vi "Autonomous A2 left-deliverswitch-move out of way.vi"   [LabVIEW 2017]
uses:
  Framework/Robot Global Data.vi
types:
  T1 = typedef "Command Status Info.ctl" = cluster{"Name":string, "Status":T2, "notifier out":T3}
  T2 = typedef "Completion Status.ctl" = enum16{"Successful", "Aborted", "Incomplete"}
  T3 = typedef "Completion Notifier.ctl" = refnum<notifier>
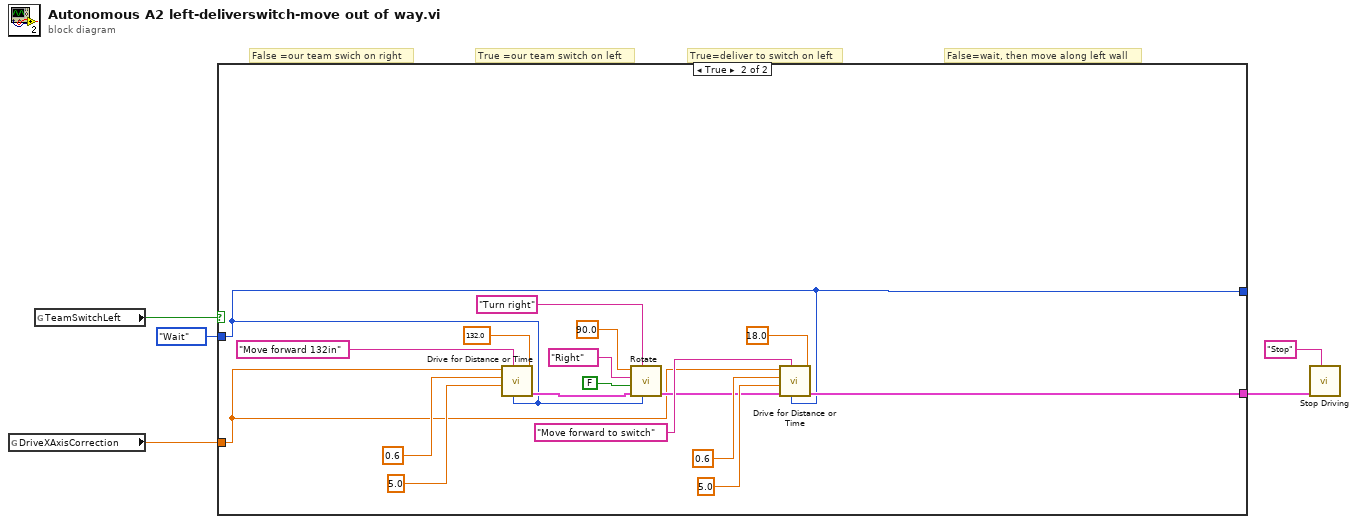
[diagram p0: block diagram]
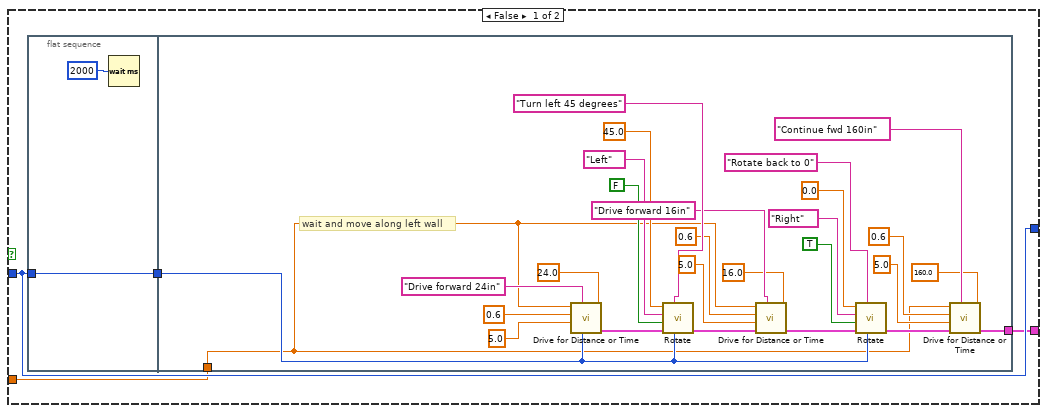
[diagram p2: hidden frame]
diagram:
  # "False=wait, then move along left wall"
  # "True=deliver to switch on left"
  # "False =our team swich on right"
  # "True =our team switch on left"
  n1 = global read "Robot Global Data.vi" "DriveXAxisCorrection"() -> (w1:dbl)
  n2 = global read "Robot Global Data.vi" "TeamSwitchLeft"() -> (w2:bool)
  n3 = case shown="True" w2 {
    tunnel: enum16{"Start", "Wait"}."Wait" ("Synchronication") -> [w9 w43]
    tunnel: [w7 w52] -> w3
    tunnel: [w9 w43] -> _
    tunnel: w1 -> [w6 w39]
    frame False {
      n4 = flat-sequence {
        tunnel: w9 -> [w11]
        tunnel: [w11] -> w8
        tunnel: w8 -> [w29]
        tunnel: [w15] -> w7
        tunnel: w6 -> [w12]
        frame #0 {
          n5 = Wait (ms)(milliseconds to wait=u32 2000) -> ()  [unwired: 1 out]
        }
        frame #1 {
          # "wait and move along left wall"
          n6 = call "Drive for Distance or Time.vi"("Distance (inches)"=24.0, "Synchronication"=w29, "Description"="Drive forward 24in", "Seconds"=5.0, "Y-axis"=0.6 ("Right Speed"), "X-axis"=w12) -> ("Command Info Out"=w35:T1)  [unwired: 5 in]
          n7 = call "Rotate.vi"("Synchronication"=w29, "Description"="Turn left 45 degrees", "Command Info In"=w35, "Force Degrees"=FALSE, "Turn Direction"="Left" ("Direction"), "Degrees"=45.0) -> ("Command Info Out"=w24:T1)  [unwired: 5 in]
          n8 = call "Drive for Distance or Time.vi"("Distance (inches)"=16.0, "Description"="Drive forward 16in", "Command Info In"=w24, "Seconds"=5.0, "Y-axis"=0.6 ("Right Speed"), "X-axis"=w12) -> ("Command Info Out"=w23:T1)  [unwired: 5 in]
          n9 = call "Rotate.vi"("Synchronication"=w29, "Description"="Rotate back to 0", "Command Info In"=w23, "Force Degrees"=TRUE, "Turn Direction"="Right" ("Direction"), "Degrees"=0.0 ("Seconds")) -> ("Command Info Out"=w22:T1)  [unwired: 5 in]
          n10 = call "Drive for Distance or Time.vi"("Distance (inches)"=160.0, "Description"="Continue fwd 160in", "Command Info In"=w22, "Seconds"=5.0, "Y-axis"=0.6, "X-axis"=w12) -> ("Command Info Out"=w15:T1)  [unwired: 5 in]
        }
      }
    }
    frame True {
      n11 = call "Drive for Distance or Time.vi"("Distance (inches)"=132.0, "Synchronication"=w43, "Description"="Move forward 132in", "Seconds"=5.0, "Y-axis"=0.6 ("Right Speed"), "X-axis"=w39) -> ("Command Info Out"=w48:T1)  [unwired: 5 in]
      n12 = call "Rotate.vi"("Synchronication"=w43, "Description"="Turn right", "Command Info In"=w48, "Force Degrees"=FALSE, "Turn Direction"="Right" ("Direction"), "Degrees"=90.0 ("Seconds")) -> ("Command Info Out"=w47:T1)  [unwired: 5 in]
      n13 = call "Drive for Distance or Time.vi"("Distance (inches)"=18.0, "Synchronication"=w43, "Description"="Move forward to switch", "Command Info In"=w47, "Seconds"=5.0, "Y-axis"=0.6 ("Right Speed"), "X-axis"=w39) -> ("Command Info Out"=w52:T1)  [unwired: 4 in]
    }
  }
  n14 = call "Stop Driving.vi"("Description"="Stop", "Command Info In"=w3) -> ()  [unwired: 9 in, 1 out]
